vi "pr2.vi"() -> ()   [LabVIEW 2014]
uses:
  <vilib>/measure/NI_MABase.lvlib
panel:
  in  "R":dbl(slide)=500.0 min=10.0 max=100000.0 step=1.0 scale=10.0..100000.0 scale format="%#.6p"
  in  "C":dbl(slide)=2e-06 min=1e-06 max=0.001 step=1e-07 scale=1e-06..0.001 scale format="%#.6p"
  in  "V":dbl(slide)=10.0 caption="Signal Voltage (V)" min=0.0 max=20.0 step=0.1 scale=0.0..20.0 scale format="%#.6p"
  in  "Frequency":dbl(slide)=50.0 caption="Signal Frequency (Hz)" min=0.0 max=500.0 step=1.0 scale=0.0..100.0 scale format="%#.6p"
  in  "DutyCycle":dbl(slide)=50.0 caption="Duty Cycle (%)" min=0.0 max=100.0 step=1.0 scale=0.0..100.0 scale format="%#.6p"
  in  "L":dbl(slide)=2e-06 min=1e-06 max=0.001 step=1e-07 scale=1e-06..0.001 scale format="%#.6p"
  out "Current Graph":waveform(dbl)[](graph)
  out "Voltage Graph":waveform(dbl)[](graph)
  out "Control Signal":waveform(dbl)[](graph)
  in  "stop":bool
  # "PSI3214"
  # "Laboratório de \nInstrumentação Elétrica"
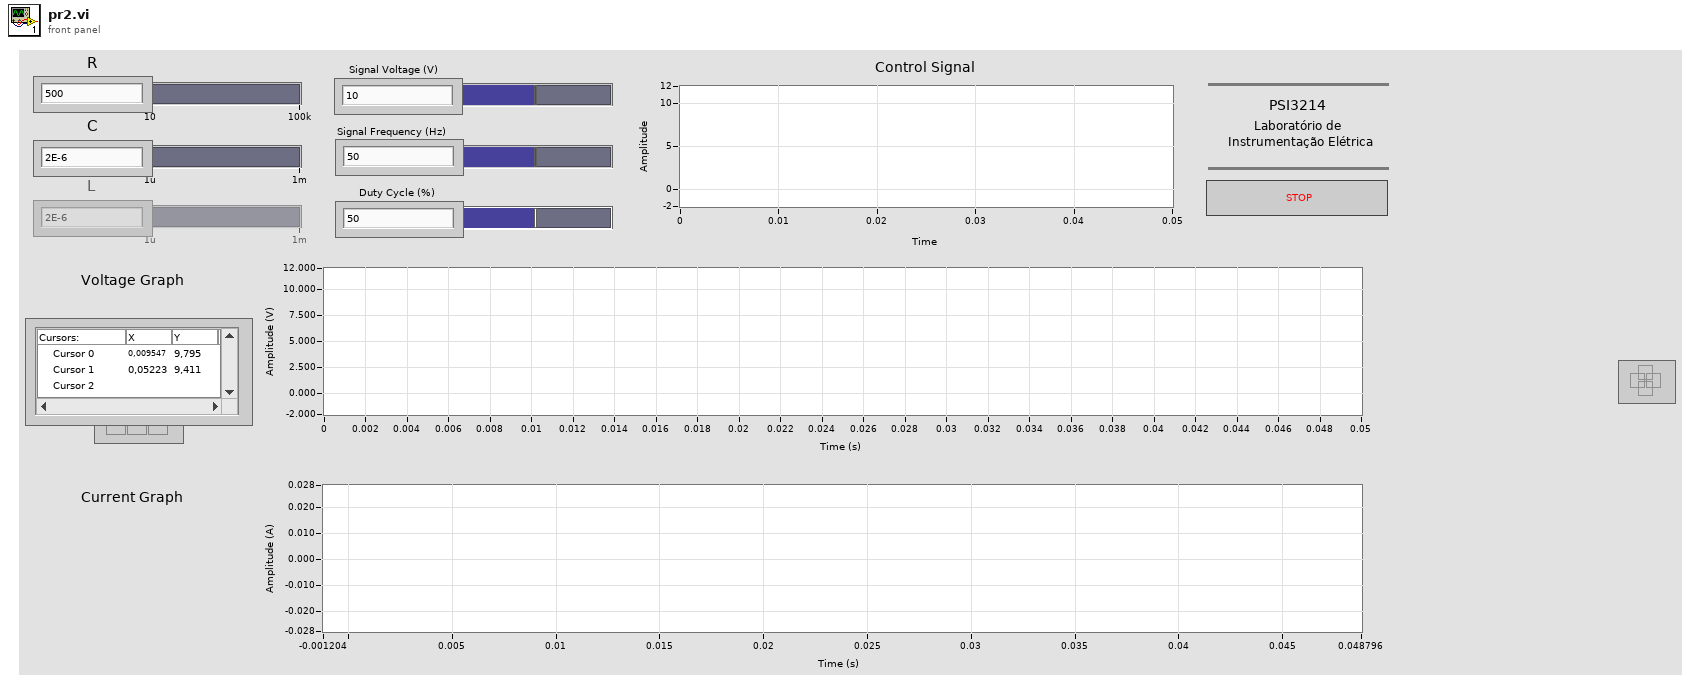
[diagram p1: front panel]
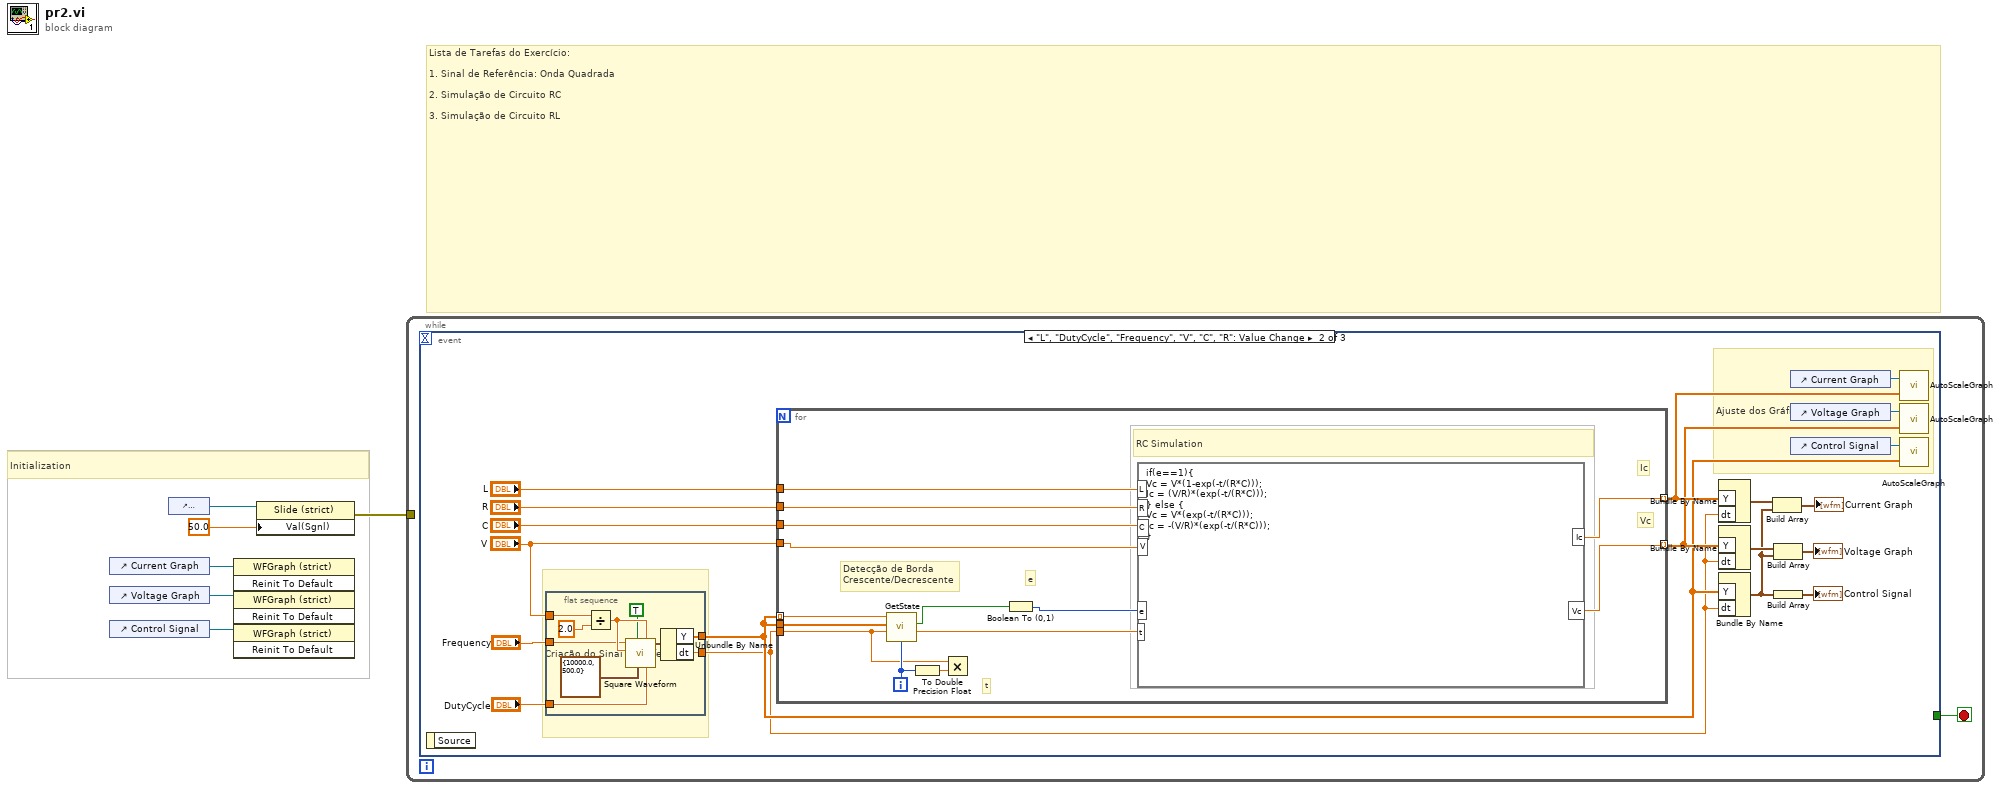
[diagram p0: block diagram]
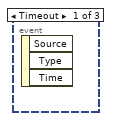
[diagram p2: hidden frame]
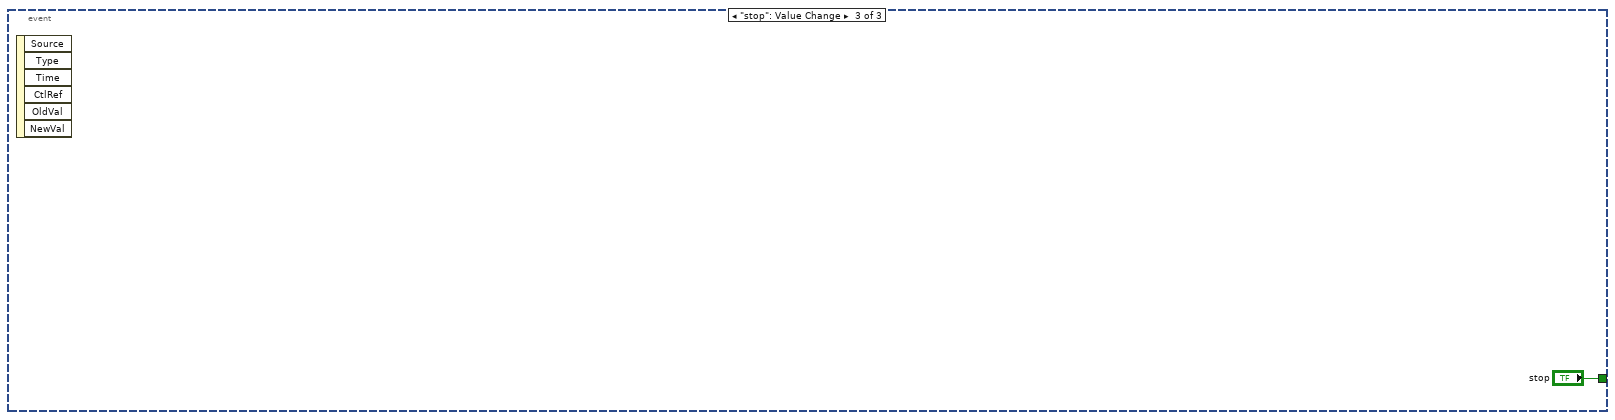
[diagram p3: hidden frame]
diagram:
  # "Initialization"
  # "Lista de Tarefas do Exercício:\n\n1. Sinal de Referência: Onda Quadrada\n\n2. Simulação de Circuito RC\n\n3. Simulação de Circuito RL"
  n1 = control-ref of="Current Graph"() -> (w4:refnum<vi>)
  n2 = control-ref of="Voltage Graph"() -> (w3:refnum<vi>)
  n3 = control-ref of="Control Signal"() -> (w2:refnum<vi>)
  n4 = control-ref of="Frequency"() -> (w1:refnum<vi>)
  n5 = invoke class="WFGraph (strict)" method="Reinit To Default"(reference=w4) -> ()  [unwired: 2 in, 3 out]
  n6 = invoke class="WFGraph (strict)" method="Reinit To Default"(reference=w3) -> ()  [unwired: 2 in, 3 out]
  n7 = invoke class="WFGraph (strict)" method="Reinit To Default"(reference=w2) -> ()  [unwired: 2 in, 3 out]
  n8 = property class="Slide (strict)"(reference=w1, "Val(Sgnl)"=50.0 ("Value (Signaling)")) -> (error out=w5:errorcluster)  [unwired: 1 in, 1 out]
  n9 = while {
    tunnel: w5 -> [_]
    stop <- w7 stop-if-true
    n10 = event shown="[1] \"L\", \"DutyCycle\", \"Frequency\", \"V\", \"C\", \"R\": Value Change" {
      selector: _ -> [_ _ _]
      dyn-events: _ -> [_ _ _]
      timeout: _ -> [_ _ _]
      tunnel: [_ _ "stop"] -> w7
      event Timeout {
        n11 = event-data() -> ()  [unwired: 1 in, 3 out]
      }
      event "L", "DutyCycle", "Frequency", "V", "C", "R": Value Change {
        # "Ajuste dos Gráficos - AutoScale"
        # "Criação do Sinal de Referencia"
        n12 = event-data() -> ()  [unwired: 1 in, 1 out]
        n13 = flat-sequence {
          tunnel: "V" -> [w32]
          tunnel: "Frequency" -> [w31]
          tunnel: "DutyCycle" -> [w30]
          tunnel: [w29] -> w15
          tunnel: [w28] -> w14
          frame #0 {
            n14 = Divide(x=w32, y=2.0) -> (x/y=w34:dbl)
            n15 = call <vilib>:"Square Waveform.vi"("duty cycle (%)"=w30, "offset"=w34, "sampling info"=cluster{"Fs":dbl, "#s":dbl} {"Fs"=10000.0, "#s"=500.0}, "reset signal"=TRUE, "amplitude"=w34, "frequency"=w31) -> ("signal out"=w33:waveform(dbl))  [unwired: 4 in, 1 out]
            n16 = Unbundle By Name(w33) -> ("Y"=w29:dbl[], "dt"=w28:dbl)
          }
        }
        n17 = for {
          tunnel: "R" -> [w42]
          tunnel: "C" -> [w41]
          tunnel: "V" -> [w40]
          tunnel: [w38] -> w19 mode=indexing
          tunnel: w15 -> [w49] mode=indexing
          tunnel: w15 -> [w50]
          tunnel: w14 -> [w45]
          tunnel: "L" -> [w43]
          tunnel: [w39] -> w22 mode=indexing
          i -> [w46]
          # "RC Simulation"
          # "Vc"
          # "Ic"
          # "t"
          # "e"
          # "Detecção de Borda\nCrescente/Decrescente"
          n18 = call "GetState.vi"("Array Element"=w49, "Array"=w50, "dt"=w45, "Loop Iteration"=w46) -> ("Rising/Falling Edge"=w48:bool, "t"=w37:dbl)  [unwired: 3 in, 1 out]
          n19 = To Double Precision Float(number=w46) -> (double precision float=w47:dbl)
          n20 = Multiply(x=w45, y=w47) -> ()  [unwired: 1 out]
          n21 = Boolean To (0,1)(Boolean=w48) -> (0, 1=w44:i16)
          n22 = formula code="if(e==1){\nVc = V*(1-exp(-t/(R*C)));\nIc = (V/R)*(exp(-t/(R*C)));\n} else {\nVc = V*(exp(-t/(R*C)));\nIc = -(V/R)*(exp(-t/(R*C)));\n}"("L"=w43, "R"=w42, "C"=w41, "V"=w40, "e"=w44, "t"=w37) -> ("Ic"=w39:dbl, "Vc"=w38:dbl)
        }
        n23 = Bundle By Name("Y"=w22, "dt"=w14) -> (w25:waveform(dbl))  [unwired: 1 in]
        n24 = Bundle By Name("Y"=w19, "dt"=w14) -> (w24:waveform(dbl))  [unwired: 1 in]
        n25 = Bundle By Name("Y"=w15, "dt"=w14) -> (w18:waveform(dbl))  [unwired: 1 in]
        n26 = Build Array(w25, w18) -> (→"Current Graph":waveform(dbl)[])
        n27 = Build Array(w24, w18) -> (→"Voltage Graph":waveform(dbl)[])
        n28 = Build Array(w18) -> (→"Control Signal":waveform(dbl)[])
        n29 = control-ref of="Current Graph"() -> (w21:refnum<vi>)
        n30 = control-ref of="Voltage Graph"() -> (w20:refnum<vi>)
        n31 = control-ref of="Control Signal"() -> (w16:refnum<vi>)
        n32 = call "AutoScaleGraph.vi"("Array"=w22, "WaveformGraph in"=w21) -> ()  [unwired: 1 in]
        n33 = call "AutoScaleGraph.vi"("Array"=w19, "WaveformGraph in"=w20) -> ()  [unwired: 1 in]
        n34 = call "AutoScaleGraph.vi"("Array"=w15, "WaveformGraph in"=w16) -> ()  [unwired: 1 in]
      }
      event "stop": Value Change {
        n35 = event-data() -> ()  [unwired: 1 in, 6 out]
      }
    }
  }
